vi "MuxSwitchSingle.vi"(7 "MUX address":u32=1 min=1 max=12 step=1, 8 "error in (no error)":errorcluster, 9 "Channel":i32=1 min=1 max=12 step=1, 10 "C1 / C2":i32=1 min=1 max=12 step=1, 11 "Switching in":refnum<class "Switching.lvclass">) -> (0 "error out":errorcluster, 2 "command string":string, 3 "Switching out":refnum<class "Switching.lvclass">)   [LabVIEW 2018, in "Switching.lvclass"]
uses:
  Switching.lvclass
  C:/ProbeTestSoftware2019/itk-strip-sensor-qc/InstrControl/InstrControl.lvclass
  MUX_CommandsGlobal.vi
  GPIBSwitching/GPIBSwitching.lvclass
  InstrControl.lvclass
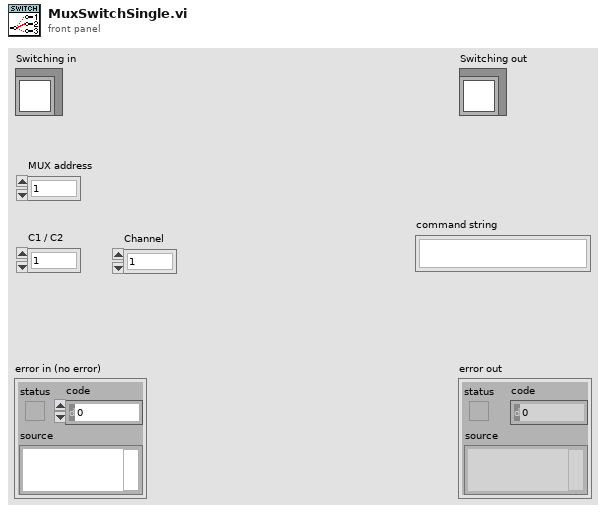
[diagram p1: front panel]
types:
  T1 = cluster{"Mux1 address":string, "Mux2 address":string, "Instrument name":string, "Instrument type":u16, "Command \"MUX Reset\"":string, "Command \"Select MUX Channel\"":string}
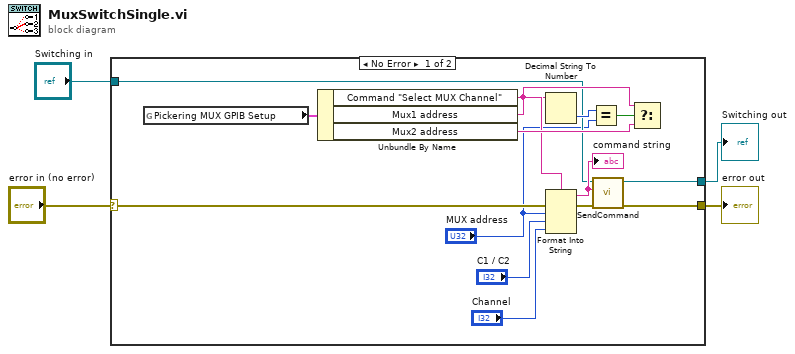
[diagram p0: block diagram]
diagram:
  n1 = case shown="No Error" "error in (no error)" {
    selector: "error in (no error)" -> [w9 w21]
    tunnel: [w7 w21] -> w3
    tunnel: [w6 w20] -> w1
    tunnel: "Switching in" -> [w8 w20]
    frame No Error {
      n2 = global read "MUX_CommandsGlobal.vi" "Pickering MUX GPIB Setup"() -> (w19:T1)
      n3 = Unbundle By Name(w19) -> ("Command \"Select MUX Channel\""=w17:string, "Mux1 address"=w11:string, "Mux2 address"=w18:string)
      n4 = Decimal String To Number(string=w11) -> (number=w12:i32)  [unwired: 2 in, 1 out]
      n5 = Format Into String(format string=w17, error in=w9, "MUX address", "C1 / C2", "Channel") -> (resulting string=w15:string, error out=w16:errorcluster)  [unwired: 1 in]
      "command string" <- w15
      n6 = Equal?(x=w12, y="MUX address") -> (x = y?=w10:bool)
      n7 = call "SendCommand.vi"("error in (no error)"=w16, "Command string"=w15, "InstControl in"=w8) -> ("error out"=w7:errorcluster, "InstControl out"=w6:refnum<class "Switching.lvclass">)  [unwired: 7 in]
      n8 = Select(t=w11, s=w10, f=w18) -> ()  [unwired: 1 out]
    }
    frame Error {
    }
  }
  "error out" <- w3
  "Switching out" <- w1
